vi "game.vi"() -> ()   [LabVIEW 2017]
panel:
  out "correct?":string
  in  "guess":dbl
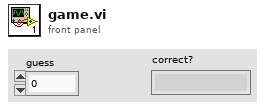
[diagram p1: front panel]
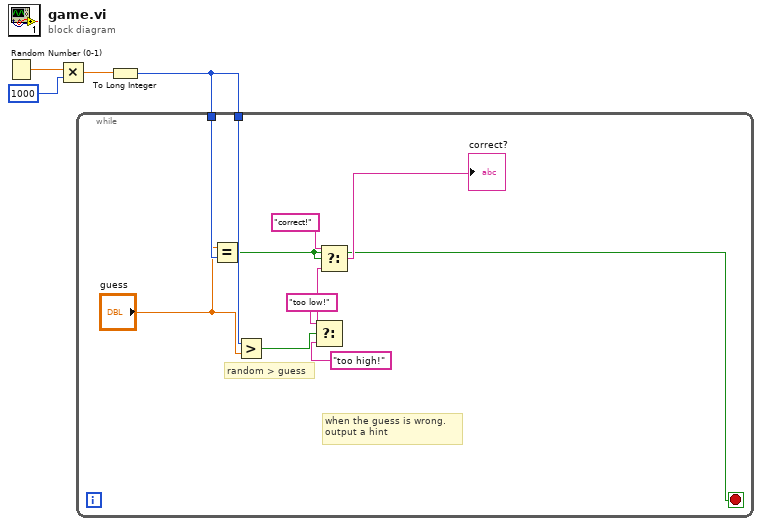
[diagram p0: block diagram]
diagram:
  n1 = Random Number (0-1)() -> (number: 0 to 1=w4:dbl)
  n2 = Multiply(x=w4, y=1000) -> (x*y=w2:dbl)
  n3 = To Long Integer(number=w2) -> (32bit integer=w1:i32)
  n4 = while {
    tunnel: w1 -> [w14]
    tunnel: w1 -> [w13]
    stop <- w5 stop-if-true
    # "random > guess"
    # "when the guess is wrong. \noutput a hint"
    n5 = Equal?(x="guess", y=w14) -> (x = y?=w5:bool)
    n6 = Greater?(x=w13, y="guess") -> (0:w11:bool)
    n7 = Select(t="too low!", s=w11, f="too high!") -> (s? t:f=w8:string)
    n8 = Select(t="correct!", s=w5, f=w8) -> (s? t:f=→"correct?":string)
  }
